vi "Autonomous Independent.vi"() -> ()   [LabVIEW 2017]
doc: "This VI is called when autonomous begins, and will automatically be terminated when autonomous ends. You can carry out timed or sensor driven robot movement independently without needing to return to the caller."
uses:
  <vilib>/Rock Robotics/WPI/SafetyOutput/WPI_SafetyOutputConfigMenu.ctl
  <vilib>/Rock Robotics/WPI/ThirdParty/Phoenix-LabVIEW/Motor Controller/Controls/CTRE_Phoenix_MotorControl_ControlMode.ctl
  Robot Global Data.vi
  <vilib>/Rock Robotics/WPI/Solenoid/Deprecated/WPI_SolenoidSetBool.vi
  <vilib>/Rock Robotics/WPI/Solenoid/Deprecated/WPI_SolenoidGetBool.vi
  <vilib>/Rock Robotics/Network Tables/NT Write String.vi
  <vilib>/Rock Robotics/Network Tables/NT Write Number.vi
panel:
  out "Source Auto":string="Left Scale"
  in  "Manual Input 2D":string[][](array[string])=[["Mid Switch Old", "L", "LR", "", "A0,T43,M4000,L2", "A0,T0,C0.5,L2", "L4", "S", "", "", "", "", "", "", ""], ["Mid Switch Old", "R", "LR", "", "A0,T-32,M4275,L2", "A0,T0,C0.5,L2", "L4", "S", "", "", "", "", "", "", ""], ["Drive Forward", "LR", "LR", "", "A0,T0,M5000", "S", "", "", "", "", "", "", "", "", ""], ["Left Scale Only", "LR", "L", "", "A90,B90,T-4,M14700", "A90,T-90,C-0.65", "A90,L3", "A90,T-90,M1500,L3", "L4", "S", "", "", "", "", ""], ["Right Scale Only", "LR", "R", "", "A-90,B-90,T-4,M14700", "A-90,T90,C-0.65", "A-90,L3", "A-90,T90,M1500,L3", "L4", "S", "", "", "", "", ""], ["Left Scale Only", "LR", "R", "Left Drive Forward", "S", "", "", "", "", "", "", "", "", "", ""], ["Right Scale Only", "LR", "L", "Right Drive Forward", "S", "", "", "", "", "", "", "", "", "", ""], ["Left Switch", "L", "LR", "", "A90,B90", "A90,T0,M6750,L2", "A90,T-90,C0.65,L2", "L4", "S", "", "", "", "", "", ""], ["Left Switch", "R", "LR", "Left Drive Forward", "S", "", "", "", "", "", "", "", "", "", ""], ["Right Switch", "R", "LR", "", "A-90,B-90", "A-90,T0,M6750,L2", "A-90,T90,C0.65,L2", "L4", "S", "", "", "", "", "", ""], ["Right Switch", "L", "LR", "Right Drive Forward", "S", "", "", "", "", "", "", "", "", "", ""], ["Left Switch or Scale", "LR", "L", "Left Scale", "S", "", "", "", "", "", "", "", "", "", ""], ["Left Switch or Scale", "L", "R", "Left Switch", "S", "", "", "", "", "", "", "", "", "", ""], ["Left Switch or Scale", "R", "R", "Left Cross Park", "S", "", "", "", "", "", "", "", "", "", ""], ["Right Switch or Scale", "LR", "R", "Right Scale", "S", "", "", "", "", "", "", "", "", "", ""], ["Right Switch or Scale", "R", "L", "Right Switch", "S", "", "", "", "", "", "", "", "", "", ""], ["Right Switch or Scale", "L", "L", "Right Cross Park", "S", "", "", "", "", "", "", "", "", "", ""], ["Mid Switch", "L", "LR", "", "A0,T43,M4350,L2", "A0,T0,C0.65,L2", "L4", "A0,T43,M-3800", "A0,T0,M1300,L1", "A0,T85,M2000,L2", "A0,T0,C0.65,L2", "L4", "A0,T0,M-2000", "S", ""], ["Mid Switch", "R", "LR", "", "A0,T-29,M4275,L2", "A0,T0,C0.65,L2", "L4", "A0,T-36,M-4200", "A0,T0,M1600,L1", "A0,T-85,M2000,L2", "A0,T0,C0.65,L2", "L4", "A0,T0,M-2000", "S", ""], ["Left Drive Forward", "LR", "LR", "", "A90,B90,T0,M5000", "S", "", "", "", "", "", "", "", "", ""], ["Right Drive Forward", "LR", "LR", "", "A-90,B-90,T0,M5000", "S", "", "", "", "", "", "", "", "", ""], ["Right Cross Park", "L", "L", "", "A-90,B-90,T0,M10400", "A25,T0,M0", "A25,T85,M4000", "S", "", "", "", "", "", "", ""], ["Right Cross Scale", "LR", "L", "", "A-90,B-90,T0,M10400", "A25,T0,M0", "A25,T89,M9700", "A25,L3", "A25,T0,M2000,L3", "L4", "S", "", "", "", ""], ["Left Cross Scale", "LR", "R", "", "A90,B90,T0,M10400", "A-25,T0,M0", "A-25,T-89,M9700", "A-25,L3", "A-25,T0,M2000,L3", "L4", "S", "", "", "", ""], ["Left Scale", "LR", "L", "Left Scale Only", "S\nS", "", "", "", "", "", "", "", "", "", ""], ["Left Scale", "LR", "R", "Left Cross Scale", "S", "", "", "", "", "", "", "", "", "", ""], ["Right Scale", "LR", "L", "Right Cross Scale", "S", "", "", "", "", "", "", "", "", "", ""], ["Right Scale", "LR", "R", "Right Scale Only", "S", "", "", "", "", "", "", "", "", "", ""], ["Left Cross Park", "R", "R", "", "A90,B90,T0,M10400", "A-25,T0,M0", "A-25,T-89,M4000", "S", "", "", "", "", "", "", ""]]
  in  "Manual Input 1D":string[](array[string])=["Mid Switch", "L", "LR", "A0,T45,M4250,L2", "A0,T0,M800,L2", "L4", "S0", "Mid Switch", "R", "LR", "A0,T-18,M4650,L2", "L4", "S0", "Drive Forward", "LR", "LR", "A0,T0,M5000,L2", "S0"]
  in  "Use Manual 1D":bool
  out "Auto Array Ran":string[](array[string])=["Left Cross Scale", "LR", "R"]
  in  "Auto Array Offset":dbl=345.0
  in  "Frame Status":dbl=8.0
  # "Format:\nAuto Code : Switch Position : Scale Position : Reference Code : Auto Sequences for the rest of the row"
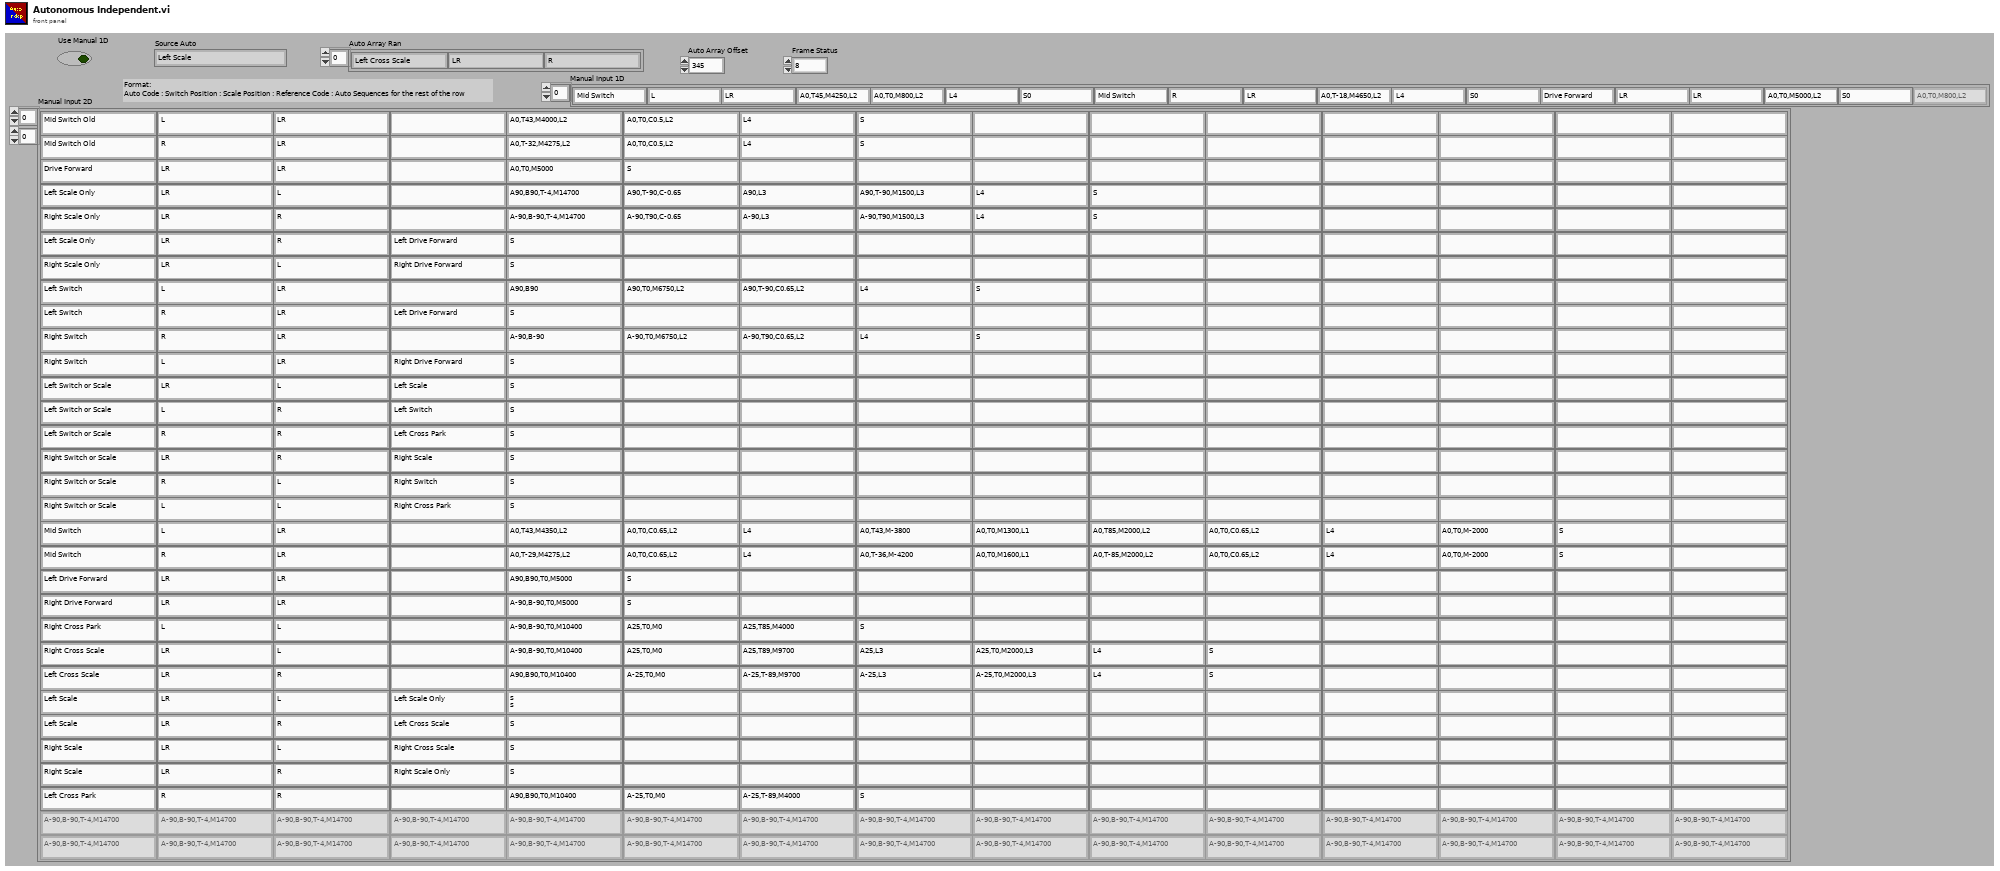
[diagram p1: front panel]
types:
  T1 = typedef "WPI_SafetyOutputConfigMenu.ctl" = enum16{"Enable", "Disable"}
  T2 = typedef "WPI_MotorControlDeviceRef.ctl" = cluster{"DeviceStatus":errorcluster, "Type":T3, "PWM":cluster{"PWM Channel":T4, "DeadBand":T5}, "CAN":cluster{"Device Number":u8, "SetOutput VI Ref":variant, "GetOutput VI Ref":variant, "Enable VI Ref":variant, "Disable VI Ref":variant, "Data":variant}, "Invert":bool, "DIO PWM":cluster{"PWM \"Enable\" Channel":T4, "DIOChannel":T6, "PWM Rate":dbl}}
  T3 = typedef "WPI_MotorControlType.ctl" = enum16{"PWM", "CAN", "DIO PWM"}
  T4 = typedef "FPGA_DIOPWMChannel.ctl" = enum8{"PWM 0", "PWM 1", "PWM 2", "PWM 3", "PWM 4", "PWM 5", "PWM 6", "PWM 7", "PWM 8", "PWM 9", "PWM MXP 0", "PWM MXP 1", "PWM MXP 2", "PWM MXP 3", "PWM MXP 4", "PWM MXP 5", "PWM MXP 6", "PWM MXP 7", "PWM MXP 8", "PWM MXP 9", "Invalid"}
  T5 = typedef "WPI_PWMDeadband.ctl" = cluster{"Name":string, "maxPositivePwm":i32, "minPositivePwm":i32, "centerPwm":i32, "maxNegativePwm":i32, "minNegativePwm":i32, "angularRange":u16}
  T6 = typedef "FPGA_DIOChannel.ctl" = enum8{"DIO 0", "DIO 1", "DIO 2", "DIO 3", "DIO 4", "DIO 5", "DIO 6", "DIO 7", "DIO 8", "DIO 9", "DIO MXP 0", "DIO MXP 1", "DIO MXP 2", "DIO MXP 3", "DIO MXP 4", "DIO MXP 5", "DIO MXP 6", "DIO MXP 7", "DIO MXP 8", "DIO MXP 9", "DIO MXP 10", "DIO MXP 11", "DIO MXP 12", "DIO MXP 13", "DIO MXP 14", "DIO MXP 15", "SPI Port CS1", "SPI Port CS2", "SPI Port CS3", "SPI Port MISO", "SPI Port MOSI", "Invalid"}
  T7 = typedef "WPI_SolenoidDevRef.ctl" = cluster{"DevStatus":errorcluster, "Pneumatics Control Module":u8, "Forward Solenoid Channel":T8, "Reverse Solenoid Channel":T8}
  T8 = typedef "WPI_SolenoidChannel.ctl" = enum8{"Solenoid 0", "Solenoid 1", "Solenoid 2", "Solenoid 3", "Solenoid 4", "Solenoid 5", "Solenoid 6", "Solenoid 7", "Invalid"}
  T9 = typedef "WPI_ServoDeviceRef.ctl" = cluster{"DeviceStatus":errorcluster, "PWM Channel":T4, "DeadBand":T5}
  T10 = typedef "CTRE_Phoenix_MotorControl_ControlMode.ctl" = u16
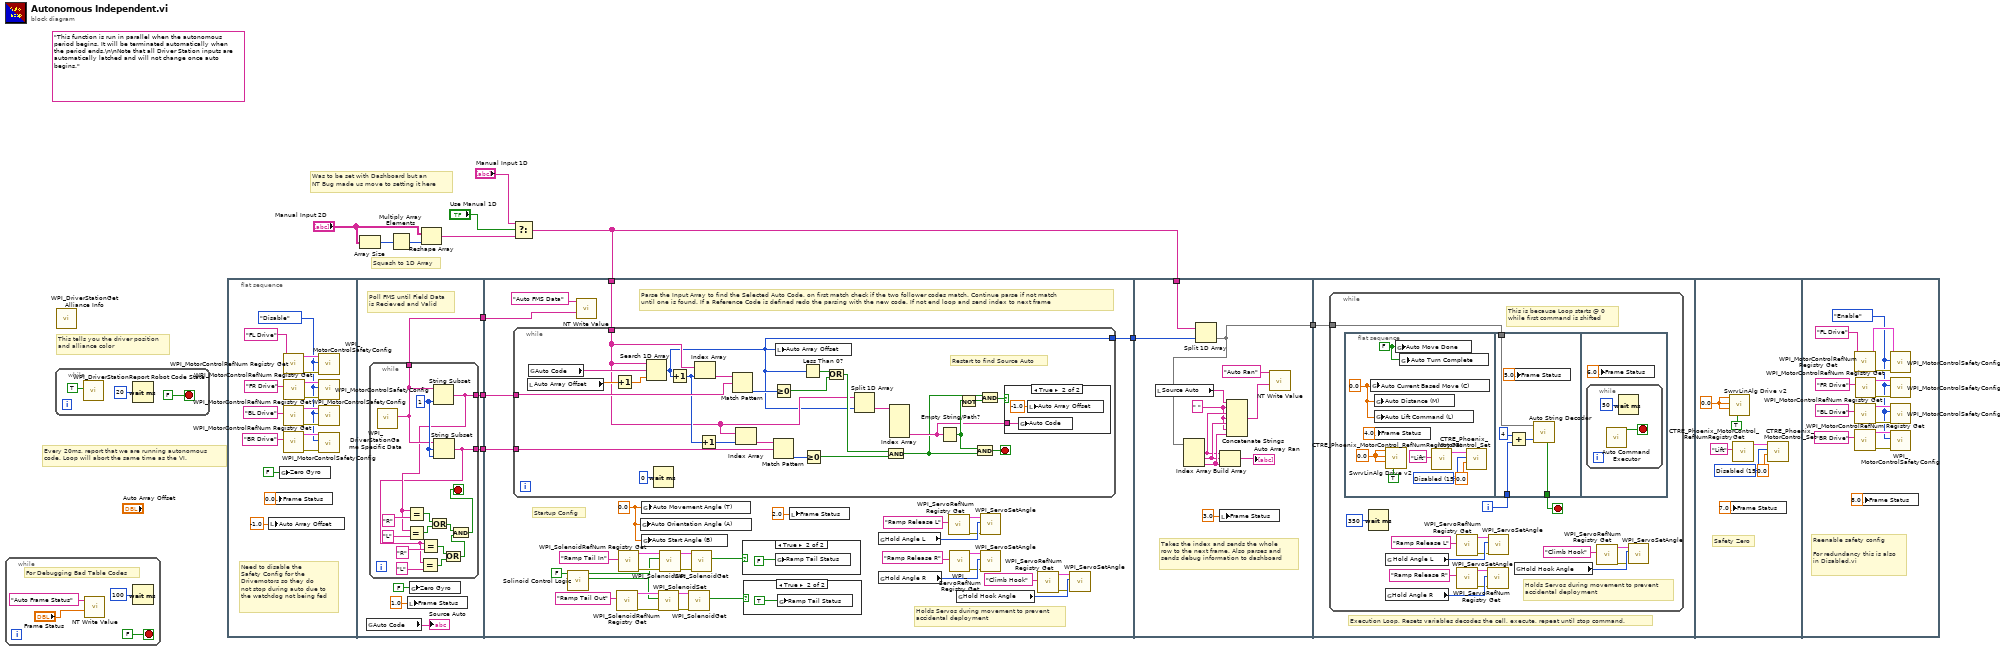
[diagram p0: block diagram]
diagram:
  (unwired) "This function is run in parallel when the autonomous period begins. It will be terminated automatically when the period ends.\n\nNote that all Driver Station inputs are automatically latched and will not change once auto begins."
  # "Was to be set with Dashboard but an\nNT Bug made us move to setting it here"
  # "Squash to 1D Array"
  # "Every 20ms, report that we are running autonomous\ncode. Loop will abort the same time as the VI."
  # "This tells you the driver position\nand alliance color"
  n1 = while {
    stop <- FALSE stop-if-true
    # "For Debugging Bad Table Codes"
    n2 = call-poly <vilib>:"NT Write Value.vi"("Numeric"="Frame Status", "Name"="Auto Frame Status") -> ()  [unwired: 9 in, 1 out]
    n3 = Wait (ms)(milliseconds to wait=u32 100) -> ()  [unwired: 1 out]
  }
  n4 = while {
    stop <- FALSE stop-if-true
    n5 = call <vilib>:"WPI_DriverStationReport Robot Code State.vi"("Autonomous"=TRUE) -> ()  [unwired: 10 in, 1 out]
    n6 = Wait (ms)(milliseconds to wait=u32 20) -> ()  [unwired: 1 out]
  }
  n7 = call <vilib>:"WPI_DriverStationGet Alliance Info.vi"() -> ()  [unwired: 12 out]
  n8 = flat-sequence {
    tunnel: [w41] -> w12
    tunnel: [w40] -> w11
    tunnel: [w38] -> w10
    tunnel: w1 -> [w91]
    tunnel: w12 -> [w89]
    tunnel: w11 -> [w88]
    tunnel: w10 -> [w87]
    tunnel: [w58] -> w6
    tunnel: w1 -> [w126]
    tunnel: [w125] -> w9
    tunnel: w6 -> [w123]
    tunnel: w9 -> [w133]
    frame #0 {
      w23 = WPI_SafetyOutputConfigMenu."Disable" ("mode")
      # "Need to disable the\nSafety Config for the\nDrivemotors so they do\nnot stop during auto due to\nthe watchdog not being fed"
      n9 = local write "Auto Array Offset"(-1.0 ("Auto Array Offset")) -> ()
      n10 = local write "Frame Status"(0.0) -> ()
      n11 = global write "Robot Global Data.vi" "Zero Gyro"(FALSE ("Zero Gyro")) -> ()
      n12 = call <vilib>:"WPI_MotorControlRefNum Registry Get.vi"("refnum name"="FL Drive") -> ("error out"=w31:errorcluster, "MotorControlDevRef"=w30:T2)  [unwired: 9 in]
      n13 = call <vilib>:"WPI_MotorControlRefNum Registry Get.vi"("refnum name"="BL Drive") -> ("error out"=w27:errorcluster, "MotorControlDevRef"=w26:T2)  [unwired: 9 in]
      n14 = call <vilib>:"WPI_MotorControlRefNum Registry Get.vi"("refnum name"="BR Drive") -> ("error out"=w25:errorcluster, "MotorControlDevRef"=w24:T2)  [unwired: 9 in]
      n15 = call <vilib>:"WPI_MotorControlRefNum Registry Get.vi"("refnum name"="FR Drive") -> ("error out"=w29:errorcluster, "MotorControlDevRef"=w28:T2)  [unwired: 9 in]
      n16 = call <vilib>:"WPI_MotorControlSafetyConfig.vi"("error in (no error)"=w31, "mode"=w23, "MotorControlDevRef"=w30) -> ()  [unwired: 7 in, 2 out]
      n17 = call <vilib>:"WPI_MotorControlSafetyConfig.vi"("error in (no error)"=w29, "mode"=w23, "MotorControlDevRef"=w28) -> ()  [unwired: 7 in, 2 out]
      n18 = call <vilib>:"WPI_MotorControlSafetyConfig.vi"("error in (no error)"=w27, "mode"=w23, "MotorControlDevRef"=w26) -> ()  [unwired: 7 in, 2 out]
      n19 = call <vilib>:"WPI_MotorControlSafetyConfig.vi"("error in (no error)"=w25, "mode"=w23, "MotorControlDevRef"=w24) -> ()  [unwired: 7 in, 2 out]
    }
    frame #1 {
      # "Poll FMS until Field Data\nis Recieved and Valid"
      n20 = global read "Robot Global Data.vi" "Auto Code"() -> (→"Source Auto":string)
      n21 = while {
        tunnel: [w45] -> w41
        tunnel: [w52] -> w40
        tunnel: [w55] -> w38
        stop <- w42 stop-if-true
        w56 = 1 ("length (rest)")
        n22 = call <vilib>:"WPI_DriverStationGame Specific Data.vi"() -> ("Game Specific Data"=w55:string)  [unwired: 11 in]
        n23 = String Subset(string=w55, length (rest)=w56) -> (substring=w52:string)  [unwired: 1 in]
        n24 = Equal?(x=w52, y="L" ("regular expression")) -> (x = y?=w51:bool)
        n25 = Equal?(x=w52, y="R" ("regular expression")) -> (x = y?=w50:bool)
        n26 = Or(x=w50, y=w51) -> (x .or. y?=w44:bool)
        n27 = String Subset(string=w55, offset (0)=w56, length (rest)=w56) -> (substring=w45:string)
        n28 = Equal?(x=w45, y="L" ("regular expression")) -> (x = y?=w47:bool)
        n29 = Equal?(x=w45, y="R" ("regular expression")) -> (x = y?=w46:bool)
        n30 = Or(x=w46, y=w47) -> (x .or. y?=w43:bool)
        n31 = And(x=w44, y=w43) -> (x .and. y?=w42:bool)
      }
      n32 = local write "Frame Status"(1.0 ("Frame Status")) -> ()
      n33 = global write "Robot Global Data.vi" "Zero Gyro"(FALSE ("Zero Gyro")) -> ()
    }
    frame #2 {
      w57 = 0.0 ("Auto Movement Angle (T)")
      # "Holds Servos during movement to prevent\naccidental deployment"
      # "Startup Config"
      # "Parse the Input Array to find the Selected Auto Code, on first match check if the two follower codes match. Continue parse if not match\nuntil one is found. If a Reference Code is defined redo the parsing with the new code. If not end loop and send index to next frame"
      n34 = while {
        tunnel: w88 -> [w117]
        tunnel: w89 -> [w113]
        tunnel: w91 -> [w95]
        tunnel: [w94] -> w58
        stop <- w97 stop-if-true
        # "Restart to find Source Auto"
        n35 = local read "Auto Array Offset"() -> (w110:dbl)
        n36 = global read "Robot Global Data.vi" "Auto Code"() -> (w103:string)
        n37 = Increment(x=w110) -> (x+1=w108:dbl)
        n38 = Search 1D Array(1D array=w95, element=w103, start index (0)=w108) -> (index of element=w94:i32)
        n39 = Wait (ms)(milliseconds to wait=u32 0) -> ()  [unwired: 1 out]
        n40 = Increment(x=w94) -> (x+1=w109:i32)
        n41 = Index Array(array=w95, index=w109) -> (element=w118:string)
        n42 = Increment(x=w109) -> (x+1=w115:i32)
        n43 = Match Pattern(string=w118, regular expression=w117) -> (offset past match=w116:i32)  [unwired: 1 in, 3 out]
        n44 = Index Array(array=w95, index=w115) -> (element=w112:string)
        n45 = Greater Or Equal To 0?(x=w116) -> (x >= 0?=w105:bool)
        n46 = Match Pattern(string=w112, regular expression=w113) -> (offset past match=w114:i32)  [unwired: 1 in, 3 out]
        n47 = local write "Auto Array Offset"(w94) -> ()
        n48 = Less Than 0?(x=w94) -> (x < 0?=w106:bool)
        n49 = Greater Or Equal To 0?(x=w114) -> (x >= 0?=w111:bool)
        n50 = Or(x=w106, y=w105) -> (x .or. y?=w104:bool)
        n51 = Split 1D Array(array=w95, index=w94) -> (second subarray=w96:string[])  [unwired: 1 out]
        n52 = And(x=w104, y=w111) -> (x .and. y?=w98:bool)
        n53 = Index Array(array=w96) -> (element #4=w99:string)  [unwired: 4 in, 3 out]
        n54 = Empty String/Path?(string/path=w99) -> (empty?=w100:bool)
        n55 = Not(x=w100) -> (.not. x?=w101:bool)
        n56 = And(x=w100, y=w98) -> (x .and. y?=w97:bool)
        n57 = And(x=w98, y=w101) -> (x .and. y?=w102:bool)
        n58 = case shown="True" w102 {
          tunnel: w99 -> [_ w120]
          frame False {
          }
          frame True {
            n59 = global write "Robot Global Data.vi" "Auto Code"(w120) -> ()
            n60 = local write "Auto Array Offset"(-1.0 ("Auto Array Offset")) -> ()
          }
        }
      }
      n61 = call "Solinoid Control Logic.vi"("Input"=FALSE) -> ("Out"=w72:bool, "In"=w73:bool)  [unwired: 9 in]
      n62 = call-poly <vilib>:"NT Write Value.vi"("String"=w87, "Name"="Auto FMS Data") -> ()  [unwired: 9 in, 1 out]
      n63 = call <vilib>:"WPI_SolenoidRefNum Registry Get.vi"("refnum name"="Ramp Tail Out") -> ("error out"=w81:errorcluster, "SolenoidDevRef"=w80:T7)  [unwired: 9 in]
      n64 = call <vilib>:"WPI_SolenoidRefNum Registry Get.vi"("refnum name"="Ramp Tail In") -> ("error out"=w83:errorcluster, "SolenoidDevRef"=w82:T7)  [unwired: 9 in]
      n65 = global write "Robot Global Data.vi" "Auto Orientation Angle (A)"(w57) -> ()
      n66 = global write "Robot Global Data.vi" "Auto Start Angle (B)"(w57) -> ()
      n67 = global write "Robot Global Data.vi" "Auto Movement Angle (T)"(w57) -> ()
      n68 = call-poly <vilib>:"WPI_SolenoidSet.vi"("error in (no error)"=w81, "Value"=w72, "SolenoidDevRef"=w80) -> ("error out"=w77:errorcluster, "SolenoidDevRef"=w76:T7)  [unwired: 7 in]
      n69 = call-poly <vilib>:"WPI_SolenoidSet.vi"("error in (no error)"=w83, "Value"=w73, "SolenoidDevRef"=w82) -> ("error out"=w79:errorcluster, "SolenoidDevRef"=w78:T7)  [unwired: 7 in]
      n70 = call-poly <vilib>:"WPI_SolenoidGet.vi"("error in (no error)"=w77, "SolenoidDevRef"=w76) -> ("Value"=w75:bool)  [unwired: 7 in, 2 out]
      n71 = call-poly <vilib>:"WPI_SolenoidGet.vi"("error in (no error)"=w79, "SolenoidDevRef"=w78) -> ("Value"=w74:bool)  [unwired: 7 in, 2 out]
      n72 = case shown="True" w74 {
        frame False {
        }
        frame True {
          n73 = global write "Robot Global Data.vi" "Ramp Tail Status"(FALSE ("Intake Short Status")) -> ()
        }
      }
      n74 = case shown="True" w75 {
        frame False {
        }
        frame True {
          n75 = global write "Robot Global Data.vi" "Ramp Tail Status"(TRUE ("Intake Short Status")) -> ()
        }
      }
      n76 = local write "Frame Status"(2.0 ("Frame Status")) -> ()
      n77 = global read "Robot Global Data.vi" "Hold Angle L"() -> (w68:i32)
      n78 = global read "Robot Global Data.vi" "Hold Angle R"() -> (w69:i32)
      n79 = call <vilib>:"WPI_ServoRefNum Registry Get.vi"("refnum name"="Ramp Release L") -> ("error out"=w62:errorcluster, "ServoDeviceRef"=w63:T9)  [unwired: 9 in]
      n80 = call <vilib>:"WPI_ServoRefNum Registry Get.vi"("refnum name"="Ramp Release R") -> ("error out"=w65:errorcluster, "ServoDeviceRef"=w64:T9)  [unwired: 9 in]
      n81 = global read "Robot Global Data.vi" "Hold Hook Angle"() -> (w70:i32)
      n82 = call <vilib>:"WPI_ServoSetAngle.vi"("error in (no error)"=w62, "Angle"=w68, "ServoDeviceRef"=w63) -> ()  [unwired: 7 in, 2 out]
      n83 = call <vilib>:"WPI_ServoSetAngle.vi"("error in (no error)"=w65, "Angle"=w69, "ServoDeviceRef"=w64) -> ()  [unwired: 7 in, 2 out]
      n84 = call <vilib>:"WPI_ServoRefNum Registry Get.vi"("refnum name"="Climb Hook") -> ("error out"=w66:errorcluster, "ServoDeviceRef"=w67:T9)  [unwired: 9 in]
      n85 = call <vilib>:"WPI_ServoSetAngle.vi"("error in (no error)"=w66, "Angle"=w70, "ServoDeviceRef"=w67) -> ()  [unwired: 7 in, 2 out]
    }
    frame #3 {
      w122 = " " ("string")
      # "Takes the index and sends the whole\nrow to the next frame. Also parses and\nsends debug information to dashboard"
      n86 = local read "Source Auto"() -> (w121:string)
      n87 = Split 1D Array(array=w126, index=w123) -> (second subarray=w125:string[])  [unwired: 1 out]
      n88 = Index Array(array=w125) -> (element #1=w130:string, element #2=w131:string, element #3=w132:string)  [unwired: 3 in]
      n89 = Build Array(w130, w131, w132) -> (→"Auto Array Ran":string[])
      n90 = local write "Frame Status"(3.0 ("Frame Status")) -> ()
      n91 = Concatenate Strings(w121, w122, w130, w122, w131, w122, w132) -> (w129:string)
      n92 = call-poly <vilib>:"NT Write Value.vi"("String"=w129, "Name"="Auto Ran") -> ()  [unwired: 9 in, 1 out]
    }
    frame #4 {
      # "Execution Loop, Resets variables decodes the cell, execute, repeat until stop command."
      n93 = while {
        tunnel: w133 -> [w135]
        i -> [w149]
        stop <- w148 stop-if-true
        # "Holds Servos during movement to prevent\naccidental deployment"
        # "This is because Loop starts @ 0 \nwhile first command is shifted"
        n94 = flat-sequence {
          tunnel: w149 -> [w164]
          tunnel: [w163] -> w148
          tunnel: w135 -> [w162]
          frame #0 {
            w150 = FALSE ("Auto Move Done")
            w154 = T10 15 items=["PercentOutput"=0, "Position"=1, "Velocity"=2, "Current"=3, "Follower"=5, "MotionProfile"=6, "MotionMagic"=7, "MotionMagicArc"=8, "MotionProfileArc"=10, "Disabled"=15] ("Control Mode")
            w157 = 0.0 ("X")
            w151 = 0.0 ("Auto Movement Angle (T)")
            n95 = global write "Robot Global Data.vi" "Auto Current Based Move (C)"(w151) -> ()
            n96 = local write "Frame Status"(4.0) -> ()
            n97 = global write "Robot Global Data.vi" "Auto Distance (M)"(w151) -> ()
            n98 = global write "Robot Global Data.vi" "Auto Lift Command (L)"(w151) -> ()
            n99 = call "SwrvLinAlg Drive v2.vi"("Auto Controls"=TRUE, "Z"=w157, "Y"=w157, "X"=w157) -> ()  [unwired: 8 in]
            n100 = global write "Robot Global Data.vi" "Auto Move Done"(w150) -> ()
            n101 = global write "Robot Global Data.vi" "Auto Turn Complete"(w150) -> ()
            n102 = call "CTRE_Phoenix_MotorControl_RefNumRegistryGet.vi"("refnum name"="Lift") -> ("PhoenixMotorControlDevRef"=w156:T2)  [unwired: 9 in, 1 out]
            n103 = call <vilib>:"CTRE_Phoenix_MotorControl_Set.vi"("Output"=0.0, "Control Mode"=w154, "PhoenixMotorControlDevRef"=w156) -> ()  [unwired: 7 in, 2 out]
          }
          frame #1 {
            n104 = Add(x=4, y=w164) -> (x+y=w161:i32)
            n105 = local write "Frame Status"(5.0) -> ()
            n106 = call "Auto String Decoder.vi"("Index"=w161, "subarray"=w162) -> ("Done with Auto"=w163:bool)  [unwired: 9 in]
          }
          frame #2 {
            n107 = while {
              stop <- w167 stop-if-true
              n108 = call "Auto Command Executor.vi"() -> ("Done Executing Command"=w167:bool)  [unwired: 11 in]
              n109 = Wait (ms)(milliseconds to wait=u32 50) -> ()  [unwired: 1 out]
            }
            n110 = local write "Frame Status"(6.0) -> ()
          }
        }
        n111 = Wait (ms)(milliseconds to wait=u32 350) -> ()  [unwired: 1 out]
        n112 = global read "Robot Global Data.vi" "Hold Angle R"() -> (w146:i32)
        n113 = global read "Robot Global Data.vi" "Hold Angle L"() -> (w145:i32)
        n114 = call <vilib>:"WPI_ServoRefNum Registry Get.vi"("refnum name"="Ramp Release L") -> ("error out"=w139:errorcluster, "ServoDeviceRef"=w140:T9)  [unwired: 9 in]
        n115 = call <vilib>:"WPI_ServoRefNum Registry Get.vi"("refnum name"="Ramp Release R") -> ("error out"=w142:errorcluster, "ServoDeviceRef"=w141:T9)  [unwired: 9 in]
        n116 = call <vilib>:"WPI_ServoSetAngle.vi"("error in (no error)"=w142, "Angle"=w146, "ServoDeviceRef"=w141) -> ()  [unwired: 7 in, 2 out]
        n117 = call <vilib>:"WPI_ServoSetAngle.vi"("error in (no error)"=w139, "Angle"=w145, "ServoDeviceRef"=w140) -> ()  [unwired: 7 in, 2 out]
        n118 = global read "Robot Global Data.vi" "Hold Hook Angle"() -> (w147:i32)
        n119 = call <vilib>:"WPI_ServoRefNum Registry Get.vi"("refnum name"="Climb Hook") -> ("error out"=w143:errorcluster, "ServoDeviceRef"=w144:T9)  [unwired: 9 in]
        n120 = call <vilib>:"WPI_ServoSetAngle.vi"("error in (no error)"=w143, "Angle"=w147, "ServoDeviceRef"=w144) -> ()  [unwired: 7 in, 2 out]
      }
    }
    frame #5 {
      w170 = T10 15 items=["PercentOutput"=0, "Position"=1, "Velocity"=2, "Current"=3, "Follower"=5, "MotionProfile"=6, "MotionMagic"=7, "MotionMagicArc"=8, "MotionProfileArc"=10, "Disabled"=15] ("Control Mode")
      w173 = 0.0 ("X")
      # "Safety Zero"
      n121 = local write "Frame Status"(7.0) -> ()
      n122 = call "SwrvLinAlg Drive v2.vi"("Auto Controls"=TRUE, "Z"=w173, "Y"=w173, "X"=w173) -> ()  [unwired: 8 in]
      n123 = call "CTRE_Phoenix_MotorControl_RefNumRegistryGet.vi"("refnum name"="Lift") -> ("PhoenixMotorControlDevRef"=w172:T2)  [unwired: 9 in, 1 out]
      n124 = call <vilib>:"CTRE_Phoenix_MotorControl_Set.vi"("Output"=0.0, "Control Mode"=w170, "PhoenixMotorControlDevRef"=w172) -> ()  [unwired: 7 in, 2 out]
    }
    frame #6 {
      w176 = WPI_SafetyOutputConfigMenu."Enable" ("mode")
      # "Reenable safety config\n\nFor redundancy this is also\nin Disabled.vi"
      n125 = call <vilib>:"WPI_MotorControlRefNum Registry Get.vi"("refnum name"="FL Drive") -> ("error out"=w184:errorcluster, "MotorControlDevRef"=w183:T2)  [unwired: 9 in]
      n126 = call <vilib>:"WPI_MotorControlRefNum Registry Get.vi"("refnum name"="BL Drive") -> ("error out"=w180:errorcluster, "MotorControlDevRef"=w179:T2)  [unwired: 9 in]
      n127 = call <vilib>:"WPI_MotorControlRefNum Registry Get.vi"("refnum name"="BR Drive") -> ("error out"=w178:errorcluster, "MotorControlDevRef"=w177:T2)  [unwired: 9 in]
      n128 = call <vilib>:"WPI_MotorControlRefNum Registry Get.vi"("refnum name"="FR Drive") -> ("error out"=w182:errorcluster, "MotorControlDevRef"=w181:T2)  [unwired: 9 in]
      n129 = local write "Frame Status"(8.0) -> ()
      n130 = call <vilib>:"WPI_MotorControlSafetyConfig.vi"("error in (no error)"=w184, "mode"=w176, "MotorControlDevRef"=w183) -> ()  [unwired: 7 in, 2 out]
      n131 = call <vilib>:"WPI_MotorControlSafetyConfig.vi"("error in (no error)"=w182, "mode"=w176, "MotorControlDevRef"=w181) -> ()  [unwired: 7 in, 2 out]
      n132 = call <vilib>:"WPI_MotorControlSafetyConfig.vi"("error in (no error)"=w180, "mode"=w176, "MotorControlDevRef"=w179) -> ()  [unwired: 7 in, 2 out]
      n133 = call <vilib>:"WPI_MotorControlSafetyConfig.vi"("error in (no error)"=w178, "mode"=w176, "MotorControlDevRef"=w177) -> ()  [unwired: 7 in, 2 out]
    }
  }
  n134 = Array Size(array="Manual Input 2D") -> (size(s)=w4:i32[])
  n135 = Multiply Array Elements(1:w4) -> (0:w5:i32)
  n136 = Reshape Array("Manual Input 2D", w5) -> (w2:string[])
  n137 = Select(t="Manual Input 1D", s="Use Manual 1D", f=w2) -> (s? t:f=w1:string[])
